vi "ReadTDMSFileFromHBM&Correct&KeepTime.vi"(4 "error in (no error)":errorcluster, 5 "dossier destination":path, 6 "file path":path) -> (0 "sortie d'erreur":errorcluster, 2 "HBMWaveformsOut":waveform(dbl)[](graph))   [LabVIEW 2017]
panel:
  out "Graphe":waveform(dbl)[](graph)
  out "iteraFinal":i32
  out "TabNomFinal":string[](array[string])
  out "ChannelNames 2":string[](array[string])
  out "size(s) 3":i32
  out "WaveformComputational":waveform(dbl)[](graph)
  out "ChannelUnit 2":string[](array[string])
  out "size(s) 2":i32
  out "Unit":string
  out "Name":string
  out "ChannelUnit":string[](array[string])
  out "ChannelNames":string[](array[string])
  out "Waveform Graph 2":waveform(dbl)(graph)
  out "WaveformHardware":waveform(dbl)[](graph)
  out "size(s)":i32
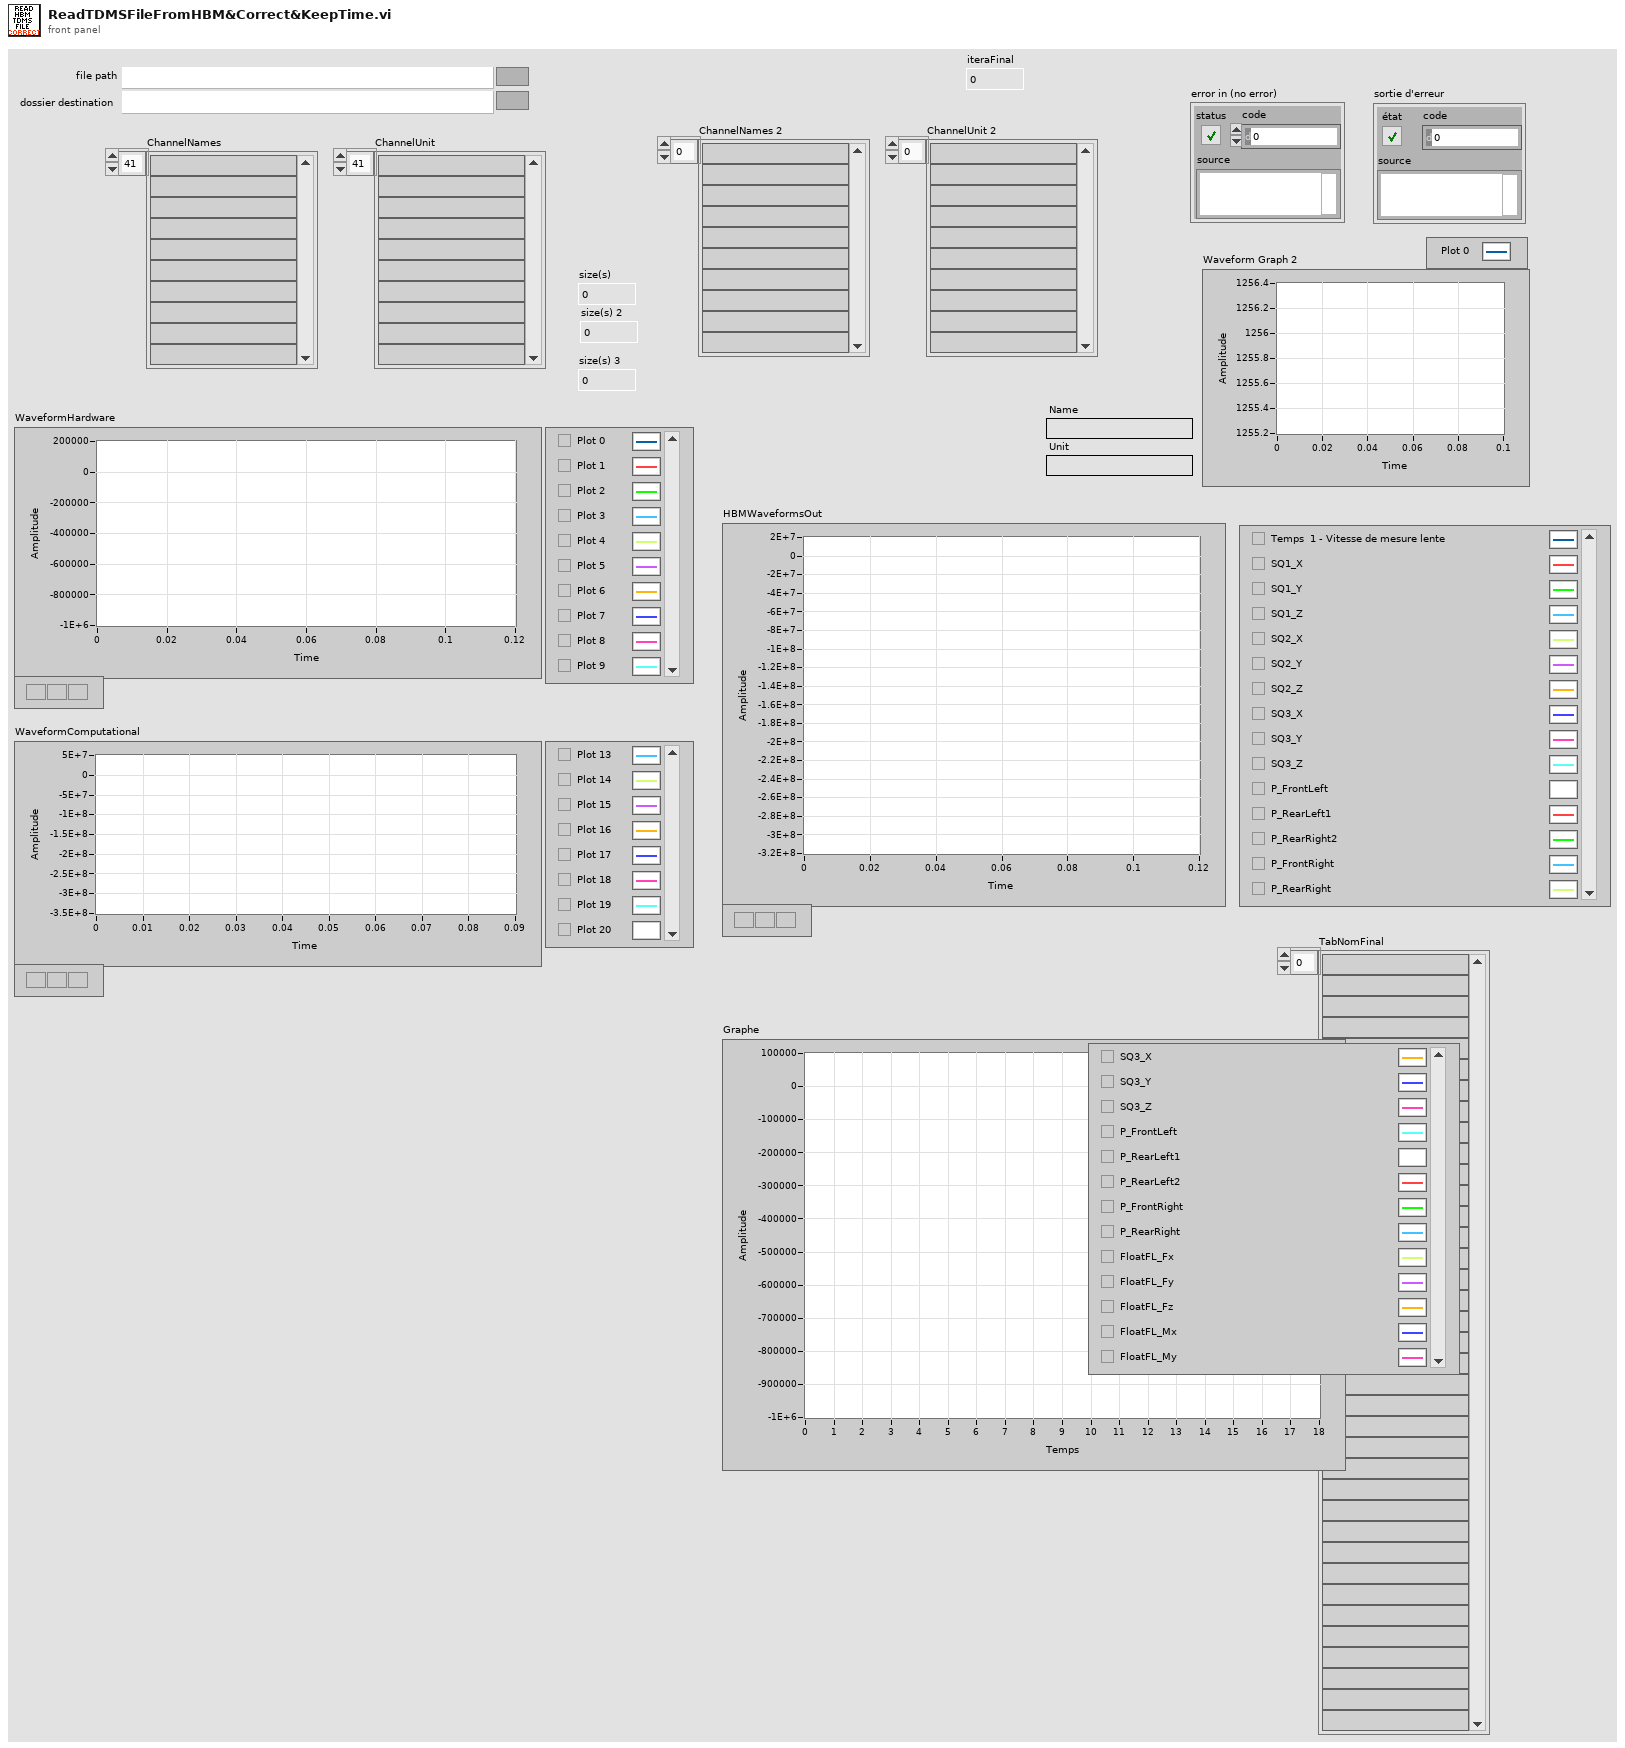
[diagram p1: front panel]
types:
  T1 = enum16{"open", "open or create", "create or replace", "create", "open (read-only)"}
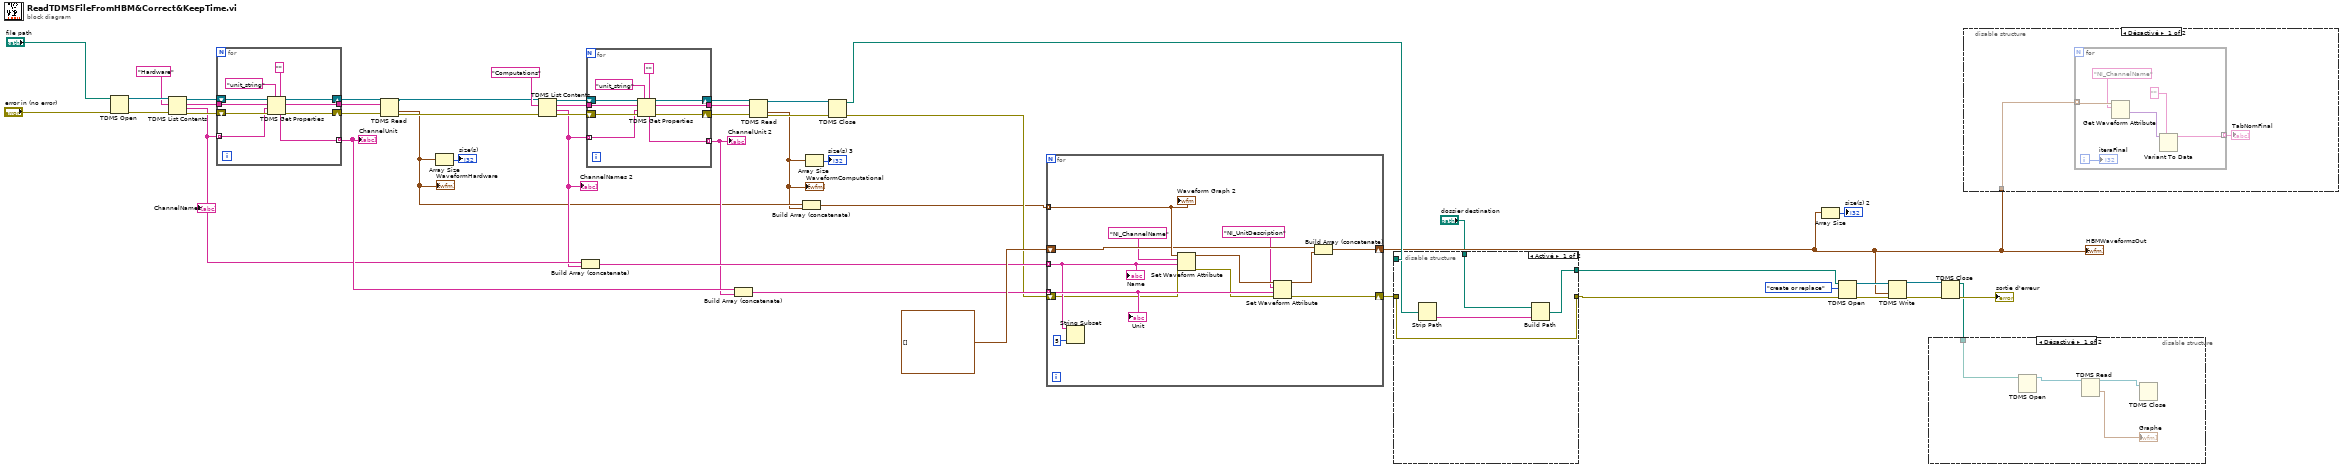
[diagram p0: block diagram]
diagram:
  n1 = TDMS Open(8:"error in (no error)", 11:"file path") -> (0:w47:errorcluster, 3:w46:refnum<k34>)  [unwired: 5 in]
  n2 = TDMS List Contents(4:w47, 6:"Hardware" ("group name"), 7:w46) -> (0:w44:errorcluster, 1:w19:string[], 2:w42:string, 3:w45:refnum<k34>)
  "ChannelNames" <- w19
  n3 = for {
    tunnel: w42 -> [w55]
    shift-right: [w57] -> w41
    shift-left: w45 -> [w59]
    shift-right: [w56] -> w40
    shift-left: w44 -> [w58]
    tunnel: w19 -> [w52] mode=indexing
    tunnel: [w51] -> w21 mode=indexing
    tunnel: [w50] -> w39
    n4 = TDMS Get Properties(5:"" ("property name"), 7:"unit_string" ("property name"), 8:w58, 9:w52, 10:w55, 11:w59) -> (0:w56:errorcluster, 2:w50:string, 3:w57:refnum<k34>, 4:w51:string)  [unwired: 2 out]
  }
  "ChannelUnit" <- w21
  n5 = TDMS Read(0:w41, 5:w39, 11:w40) -> (4:w25:refnum<k34>, 10:w17:waveform(dbl)[], 15:w26:errorcluster)  [unwired: 5 in, 3 out]
  "WaveformHardware" <- w17
  n6 = Array Size(array=w17) -> (size(s)=→"size(s)":i32)
  n7 = TDMS List Contents(4:w26, 6:"Computations" ("group name"), 7:w25) -> (0:w31:errorcluster, 1:w18:string[], 2:w33:string, 3:w30:refnum<k34>)
  "ChannelNames 2" <- w18
  n8 = Build Array (concatenate)(w19, w18) -> (w24:string[])
  n9 = for {
    tunnel: w33 -> [w65]
    shift-right: [w67] -> w34
    shift-left: w30 -> [w69]
    shift-right: [w66] -> w35
    shift-left: w31 -> [w68]
    tunnel: w18 -> [w62] mode=indexing
    tunnel: [w61] -> w20 mode=indexing
    tunnel: [w60] -> w36
    n10 = TDMS Get Properties(5:"" ("property name"), 7:"unit_string" ("property name"), 8:w68, 9:w62, 10:w65, 11:w69) -> (0:w66:errorcluster, 2:w60:string, 3:w67:refnum<k34>, 4:w61:string)  [unwired: 2 out]
  }
  "ChannelUnit 2" <- w20
  n11 = Build Array (concatenate)(w21, w20) -> (w23:string[])
  n12 = TDMS Read(0:w34, 5:w36, 11:w35) -> (4:w28:refnum<k34>, 10:w16:waveform(dbl)[], 15:w27:errorcluster)  [unwired: 5 in, 3 out]
  "WaveformComputational" <- w16
  n13 = Build Array (concatenate)(w17, w16) -> (w15:waveform(dbl)[])
  n14 = Array Size(array=w16) -> (size(s)=→"size(s) 3":i32)
  n15 = TDMS Close(8:w27, 11:w28) -> (0:w22:errorcluster, 3:w5:path)
  n16 = for {
    tunnel: w15 -> [w82] mode=indexing
    tunnel: w24 -> [w79] mode=indexing
    tunnel: w23 -> [w81] mode=indexing
    shift-right: [w77] -> w3
    shift-left: waveform(dbl)[] [] -> [w76]
    shift-right: [w80] -> w7
    shift-left: w22 -> [w75]
    n17 = String Subset(string=w79, length (rest)=5 ("length (rest)")) -> ()  [unwired: 1 in, 1 out]
    n18 = Set Waveform Attribute(4:w75, 5:w79, 6:"NI_ChannelName" ("name"), 7:w82) -> (0:w74:errorcluster, 3:w73:waveform(dbl))  [unwired: 1 out]
    n19 = Set Waveform Attribute(4:w74, 5:w81, 6:"NI_UnitDescription" ("name"), 7:w73) -> (0:w80:errorcluster, 3:w70:waveform(dbl))  [unwired: 1 out]
    n20 = Build Array (concatenate)(w76, w70) -> (w77:waveform(dbl)[])
    "Waveform Graph 2" <- w82
    "Name" <- w79
    "Unit" <- w81
  }
  "HBMWaveformsOut" <- w3
  n21 = disable-structure shown="Activé" {
    disable-tunnel: w7 -> [w83 w88]
    disable-tunnel: [w83 w88] -> w6
    disable-tunnel: w5 -> [w87 w89]
    disable-tunnel: [w86 w89] -> w4
    disable-tunnel: "dossier destination" -> [w85 _]
    frame Enabled {
      n22 = Strip Path(path=w87) -> (name=w84:string)  [unwired: 1 out]
      n23 = Build Path(base path=w85, name or relative path=w84) -> (appended path=w86:path)
    }
    frame Disabled {
    }
  }
  n24 = Array Size(array=w3) -> (size(s)=→"size(s) 2":i32)
  n25 = TDMS Open(8:w6, 10:T1."create or replace" ("opération (0 : open)"), 11:w4) -> (0:w14:errorcluster, 3:w12:refnum<k34>)  [unwired: 4 in]
  n26 = TDMS Write(0:w12, 9:w3, 11:w14) -> (4:w11:refnum<k34>, 15:w13:errorcluster)  [unwired: 3 in, 2 out]
  n27 = TDMS Close(8:w13, 11:w11) -> (0:→"sortie d'erreur":errorcluster, 3:w2:path)
  n28 = disable-structure shown="Désactivé" {
    disable-tunnel: w2 -> [w93 _]
    frame Disabled {
      n29 = TDMS Open(11:w93) -> (3:w92:refnum<k34>)  [unwired: 6 in, 1 out]
      n30 = TDMS Read(0:w92) -> (4:w91:refnum<k34>, 10:→"Graphe":waveform(dbl)[])  [unwired: 7 in, 4 out]
      n31 = TDMS Close(11:w91) -> ()  [unwired: 1 in, 2 out]
    }
    frame Enabled {
    }
  }
  n32 = disable-structure shown="Désactivé" {
    disable-tunnel: w3 -> [w95 _]
    frame Disabled {
      n33 = for {
        tunnel: w95 -> [w101] mode=indexing
        tunnel: [w97] -> w94 mode=indexing
        i -> [w96]
        n34 = Get Waveform Attribute(6:"NI_ChannelName" ("name"), 7:w101) -> (1:w99:variant)  [unwired: 2 in, 3 out]
        n35 = Variant To Data(type="" ("name"), Variant=w99) -> (data=w97:string)  [unwired: 1 in, 1 out]
        "iteraFinal" <- w96
      }
      "TabNomFinal" <- w94
    }
    frame Enabled {
    }
  }
